vi "PRIME Detector Send OPEN.vi"(8 "error in (no error)":errorcluster, 11 "connection ID":refnum<k5>) -> (0 "error out":errorcluster, 3 "connection ID out":refnum<k5>)   [LabVIEW 2024, in "PRIME Detector.lvclass"]
uses:
  PRIME Detector.lvclass
panel:
  out "Responses":string[](array[string])
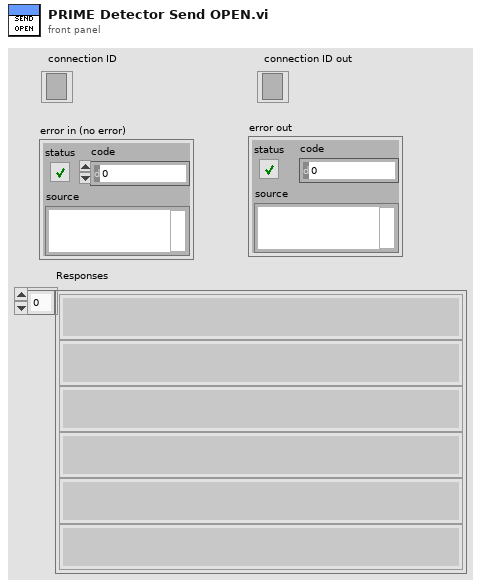
[diagram p1: front panel]
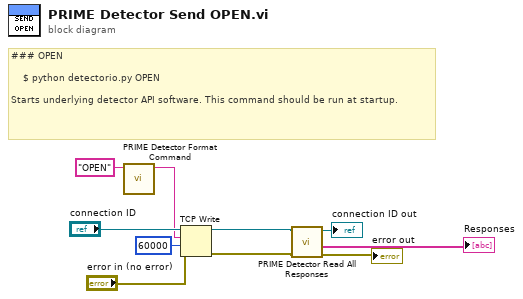
[diagram p0: block diagram]
diagram:
  # "### OPEN\n\n    $ python detectorio.py OPEN\n\nStarts underlying detector API software. This command should be run at startup."
  n1 = call "PRIME Detector Format Command.vi"("Command"="OPEN") -> ("TCP String"=w8:string)  [unwired: 10 in]
  n2 = TCP Write(connection ID="connection ID", data in=w8, error in (no error)="error in (no error)", 9:60000 ("timeout ms (25000)")) -> (connection ID out=w6:refnum<k5>, error out=w5:errorcluster)  [unwired: 1 out]
  n3 = call "PRIME Detector Read All Responses.vi"("error in"=w5, "connection ID"=w6) -> ("error out"=→"error out":errorcluster, "Responses"=→"Responses":string[], "connection ID out"=→"connection ID out":refnum<k5>)  [unwired: 6 in, 1 out]
